vi "recieveMessages.vi"(8 "error in (no error)":errorcluster, 9 "port":i32, 10 "Service":string, 11 "NetworkClient in":refnum<class "NetworkServer.lvclass">) -> (0 "error out":errorcluster, 3 "NetworkClient out":refnum<class "NetworkServer.lvclass">)   [LabVIEW 2011, in "Hardware.lvlib" / "HWControllers.lvlib" / "NetworkServer.lvclass"]
uses:
  NetworkServer.lvclass
panel:
  in  "stop":bool
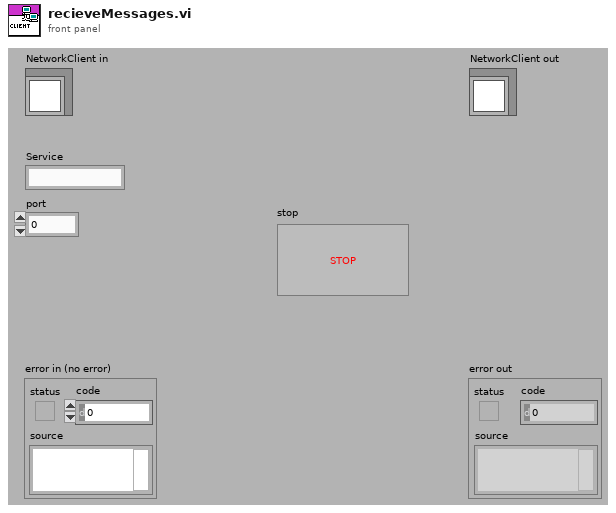
[diagram p1: front panel]
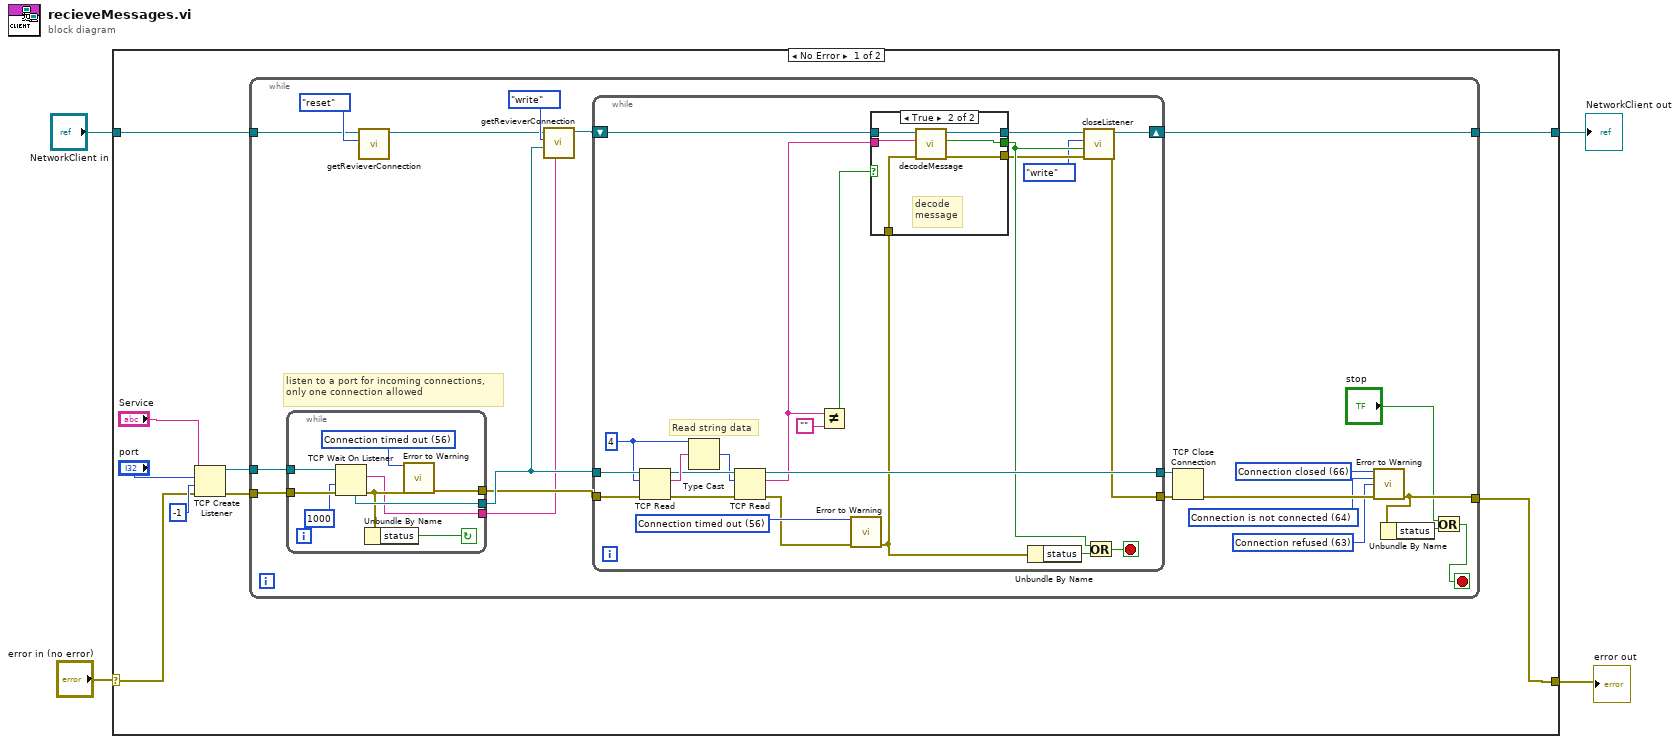
[diagram p0: block diagram]
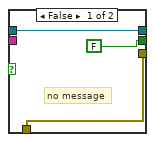
[diagram p2: hidden frame]
diagram:
  n1 = case shown="No Error" "error in (no error)" {
    selector: "error in (no error)" -> [w5 w77]
    tunnel: [w11 w77] -> w3
    tunnel: [w13 w76] -> w1
    tunnel: "NetworkClient in" -> [w12 w76]
    frame No Error {
      n2 = TCP Create Listener(8:w5, 9:-1, 10:"port", 11:"Service") -> (0:w6:errorcluster, 3:w7:refnum<k5>)  [unwired: 1 in, 1 out]
      n3 = while {
        tunnel: [w30] -> w13
        tunnel: w12 -> [w25]
        tunnel: [w17] -> w11
        tunnel: w7 -> [w22]
        tunnel: w6 -> [w20]
        stop <- w14 stop-if-true
        w23 = 63 items=["No Error", "Argument Error", "Memory Full", "Out of Zone", "End of File", "File Already Open", "Generic File IO Error", "File Not Found", "File Permission Error", "Disk Full", "Duplicate Path", "Too Many Files Open", "Not Enabled", "Resource File Not Found", "Cannot Add Resource", "Resource Not Found", "Image Not Found", "Image Memory Error", "Pen Does Not Exist", "Config Bad Type", "Config Token Not Found", "Config Parse Error", "Config Memory Error", "Bad External Code Format", "Bad External Code Offset", "External Code Not Present", "Null Window", "Destroy Window Mixup", "Null Menu", "Print Aborted", "Bad Print Record", "Print Driver Error", "Windows Error During Print", "Memory Error During Print", "Print Dialog Error", "Generic Print Error", "Invalid Device Refnum", "Device Not Found", "Device Parameter Error", "Device Unit Error", "Can't Open Device", "Device Call Aborted", "Generic Error", "Cancelled By User", "Object ID Too Low", "Object ID Too High", "Object Not In Heap", "Unknown Heap", "Bad DefProc ID", "DefProc Not In Table", "Message Out Of Range", "Null Method", "Unknown Message", "Manager Call Not Supported", "Bad address", "Connection In progress", "Connection timed out", "Connection is already in progress", "Network attribute not supported", "Network error", "Address in use", "System out of memory", "Connection aborted", "Connection refused", "Connection is not connected", "Connection is already connected", "Connection closed", "Initialize error (interapplication manager)", "Bad occurrence", "Wait on unbound occurrence handler", "Occurrence queue overflow", "Bad path", "Semaphore not signaled", "Unrecognized type (interapplication manager)"] ("1st Error to Convert")
        w24 = 64 items=["No Error", "Argument Error", "Memory Full", "Out of Zone", "End of File", "File Already Open", "Generic File IO Error", "File Not Found", "File Permission Error", "Disk Full", "Duplicate Path", "Too Many Files Open", "Not Enabled", "Resource File Not Found", "Cannot Add Resource", "Resource Not Found", "Image Not Found", "Image Memory Error", "Pen Does Not Exist", "Config Bad Type", "Config Token Not Found", "Config Parse Error", "Config Memory Error", "Bad External Code Format", "Bad External Code Offset", "External Code Not Present", "Null Window", "Destroy Window Mixup", "Null Menu", "Print Aborted", "Bad Print Record", "Print Driver Error", "Windows Error During Print", "Memory Error During Print", "Print Dialog Error", "Generic Print Error", "Invalid Device Refnum", "Device Not Found", "Device Parameter Error", "Device Unit Error", "Can't Open Device", "Device Call Aborted", "Generic Error", "Cancelled By User", "Object ID Too Low", "Object ID Too High", "Object Not In Heap", "Unknown Heap", "Bad DefProc ID", "DefProc Not In Table", "Message Out Of Range", "Null Method", "Unknown Message", "Manager Call Not Supported", "Bad address", "Connection In progress", "Connection timed out", "Connection is already in progress", "Network attribute not supported", "Network error", "Address in use", "System out of memory", "Connection aborted", "Connection refused", "Connection is not connected", "Connection is already connected", "Connection closed", "Initialize error (interapplication manager)", "Bad occurrence", "Wait on unbound occurrence handler", "Occurrence queue overflow", "Bad path", "Semaphore not signaled", "Unrecognized type (interapplication manager)"] ("1st Error to Convert")
        w33 = 66 items=["No Error", "Argument Error", "Memory Full", "Out of Zone", "End of File", "File Already Open", "Generic File IO Error", "File Not Found", "File Permission Error", "Disk Full", "Duplicate Path", "Too Many Files Open", "Not Enabled", "Resource File Not Found", "Cannot Add Resource", "Resource Not Found", "Image Not Found", "Image Memory Error", "Pen Does Not Exist", "Config Bad Type", "Config Token Not Found", "Config Parse Error", "Config Memory Error", "Bad External Code Format", "Bad External Code Offset", "External Code Not Present", "Null Window", "Destroy Window Mixup", "Null Menu", "Print Aborted", "Bad Print Record", "Print Driver Error", "Windows Error During Print", "Memory Error During Print", "Print Dialog Error", "Generic Print Error", "Invalid Device Refnum", "Device Not Found", "Device Parameter Error", "Device Unit Error", "Can't Open Device", "Device Call Aborted", "Generic Error", "Cancelled By User", "Object ID Too Low", "Object ID Too High", "Object Not In Heap", "Unknown Heap", "Bad DefProc ID", "DefProc Not In Table", "Message Out Of Range", "Null Method", "Unknown Message", "Manager Call Not Supported", "Bad address", "Connection In progress", "Connection timed out", "Connection is already in progress", "Network attribute not supported", "Network error", "Address in use", "System out of memory", "Connection aborted", "Connection refused", "Connection is not connected", "Connection is already connected", "Connection closed", "Initialize error (interapplication manager)", "Bad occurrence", "Wait on unbound occurrence handler", "Occurrence queue overflow", "Bad path", "Semaphore not signaled", "Unrecognized type (interapplication manager)"] ("1st Error to Convert")
        # "listen to a port for incoming connections,\nonly one connection allowed"
        n4 = while {
          tunnel: w22 -> [w43]
          tunnel: [w42] -> w21
          tunnel: w20 -> [w41]
          tunnel: [w39] -> w19
          tunnel: [w35] -> w18
          stop <- w36 continue-if-true
          w38 = 56 items=["No Error", "Argument Error", "Memory Full", "Out of Zone", "End of File", "File Already Open", "Generic File IO Error", "File Not Found", "File Permission Error", "Disk Full", "Duplicate Path", "Too Many Files Open", "Not Enabled", "Resource File Not Found", "Cannot Add Resource", "Resource Not Found", "Image Not Found", "Image Memory Error", "Pen Does Not Exist", "Config Bad Type", "Config Token Not Found", "Config Parse Error", "Config Memory Error", "Bad External Code Format", "Bad External Code Offset", "External Code Not Present", "Null Window", "Destroy Window Mixup", "Null Menu", "Print Aborted", "Bad Print Record", "Print Driver Error", "Windows Error During Print", "Memory Error During Print", "Print Dialog Error", "Generic Print Error", "Invalid Device Refnum", "Device Not Found", "Device Parameter Error", "Device Unit Error", "Can't Open Device", "Device Call Aborted", "Generic Error", "Cancelled By User", "Object ID Too Low", "Object ID Too High", "Object Not In Heap", "Unknown Heap", "Bad DefProc ID", "DefProc Not In Table", "Message Out Of Range", "Null Method", "Unknown Message", "Manager Call Not Supported", "Bad address", "Connection In progress", "Connection timed out", "Connection is already in progress", "Network attribute not supported", "Network error", "Address in use", "System out of memory", "Connection aborted", "Connection refused", "Connection is not connected", "Connection is already connected", "Connection closed", "Initialize error (interapplication manager)", "Bad occurrence", "Wait on unbound occurrence handler", "Occurrence queue overflow", "Bad path", "Semaphore not signaled", "Unrecognized type (interapplication manager)"] ("1st Error to Convert")
          n5 = TCP Wait On Listener(8:w41, 9:1000, 11:w43) -> (0:w37:errorcluster, 2:w35:string, 4:w42:refnum<k5>)  [unwired: 1 in, 2 out]
          n6 = Unbundle By Name(w37) -> ("status"=w36:bool)
          n7 = call <vilib>:"Error to Warning.vi"("1st Error to Convert"=w38, "error in"=w37) -> ("warning out"=w39:errorcluster)  [unwired: 3 in, 10 out]
        }
        n8 = call "getRevieverConnection.vi"("Enum"=enum16{"read", "write", "reset"}."reset", "NetworkServer in"=w25) -> ("NetworkServer out"=w26:refnum<class "NetworkServer.lvclass">)  [unwired: 5 in, 4 out]
        n9 = call "getRevieverConnection.vi"("Remote Connection"=w18, "new client"=w21, "Enum"=enum16{"read", "write", "reset"}."write", "NetworkServer in"=w26) -> ("NetworkServer out"=w29:refnum<class "NetworkServer.lvclass">)  [unwired: 3 in, 4 out]
        n10 = while {
          tunnel: [w61] -> w32
          tunnel: w19 -> [w65]
          tunnel: w21 -> [w66]
          tunnel: [w46] -> w31
          shift-right: [w49] -> w30
          shift-left: w29 -> [w55]
          stop <- w60 stop-if-true
          w52 = 56 items=["No Error", "Argument Error", "Memory Full", "Out of Zone", "End of File", "File Already Open", "Generic File IO Error", "File Not Found", "File Permission Error", "Disk Full", "Duplicate Path", "Too Many Files Open", "Not Enabled", "Resource File Not Found", "Cannot Add Resource", "Resource Not Found", "Image Not Found", "Image Memory Error", "Pen Does Not Exist", "Config Bad Type", "Config Token Not Found", "Config Parse Error", "Config Memory Error", "Bad External Code Format", "Bad External Code Offset", "External Code Not Present", "Null Window", "Destroy Window Mixup", "Null Menu", "Print Aborted", "Bad Print Record", "Print Driver Error", "Windows Error During Print", "Memory Error During Print", "Print Dialog Error", "Generic Print Error", "Invalid Device Refnum", "Device Not Found", "Device Parameter Error", "Device Unit Error", "Can't Open Device", "Device Call Aborted", "Generic Error", "Cancelled By User", "Object ID Too Low", "Object ID Too High", "Object Not In Heap", "Unknown Heap", "Bad DefProc ID", "DefProc Not In Table", "Message Out Of Range", "Null Method", "Unknown Message", "Manager Call Not Supported", "Bad address", "Connection In progress", "Connection timed out", "Connection is already in progress", "Network attribute not supported", "Network error", "Address in use", "System out of memory", "Connection aborted", "Connection refused", "Connection is not connected", "Connection is already connected", "Connection closed", "Initialize error (interapplication manager)", "Bad occurrence", "Wait on unbound occurrence handler", "Occurrence queue overflow", "Bad path", "Semaphore not signaled", "Unrecognized type (interapplication manager)"] ("1st Error to Convert")
          w58 = 4
          # "Read string data"
          n11 = TCP Read(connection ID=w66, bytes to read=w58, error in (no error)=w65) -> (connection ID out=w62:refnum<k5>, data out=w64:string, error out=w63:errorcluster)  [unwired: 1 in, 1 out]
          n12 = Type Cast(type=w58, x=w64) -> (*(type *) &x=w57:i32)
          n13 = TCP Read(connection ID=w62, bytes to read=w57, error in (no error)=w63) -> (connection ID out=w61:refnum<k5>, data out=w53:string, error out=w51:errorcluster)  [unwired: 1 in, 1 out]
          n14 = Not Equal?(x=w53, y="") -> (x != y?=w54:bool)
          n15 = call <vilib>:"Error to Warning.vi"("1st Error to Convert"=w52, "error in"=w51) -> ("warning out"=w44:errorcluster)  [unwired: 3 in, 10 out]
          n16 = case shown="True" w54 {
            tunnel: w55 -> [w69 w75]
            tunnel: [w69 w74] -> w50
            tunnel: w44 -> [w68 w73]
            tunnel: [w68 w72] -> w47
            tunnel: w53 -> [_ w71]
            tunnel: [FALSE w70] -> w48
            frame False {
              # "no message"
            }
            frame True {
              # "decode\nmessage"
              n17 = call-dynamic "decodeMessage.vi"("error in (no error)"=w73, "MessageString"=w71, "NetworkClient in"=w75) -> ("error out"=w72:errorcluster, "close"=w70:bool, "NetworkClient out"=w74:refnum<class "NetworkServer.lvclass">)  [unwired: 6 in]
            }
          }
          n18 = Unbundle By Name(w44) -> ("status"=w59:bool)
          n19 = call "closeListener.vi"("error in (no error)"=w47, "close"=w48, "actions"=enum16{"read", "write"}."write", "NetworkServer in"=w50) -> ("error out"=w46:errorcluster, "NetworkServer out"=w49:refnum<class "NetworkServer.lvclass">)  [unwired: 5 in, 1 out]
          n20 = Or(x=w48, y=w59) -> (x .or. y?=w60:bool)
        }
        n21 = TCP Close Connection(connection ID=w32, error in (no error)=w31) -> (error out=w34:errorcluster)  [unwired: 1 in, 1 out]
        n22 = call <vilib>:"Error to Warning.vi"("1st Error to Convert"=w33, "2nd Error to Convert"=w24, "3rd Error to Convert"=w23, "error in"=w34) -> ("warning out"=w17:errorcluster)  [unwired: 1 in, 10 out]
        n23 = Unbundle By Name(w17) -> ("status"=w15:bool)
        n24 = Or(x="stop", y=w15) -> (x .or. y?=w14:bool)
      }
    }
    frame Error {
    }
  }
  "error out" <- w3
  "NetworkClient out" <- w1
